vi "BuildExperiment.vi"(0 "object in":refnum<class "Application.lvclass">, 2 "Experiment Settings":T1={"Frequencies (MHz)"=[], "Camera Settings"={"Minimum Time between\n frames(s)"=10.0, "Number of Frames"=0}, "Flowrates (ul/min)"=[], "Voltages"=[]} {"Camera Settings"."Minimum Time between\n frames(s)" min=0.005}, 5 "error in (no error)":errorcluster) -> (14 "object out":refnum<class "Application.lvclass">, 19 "error out":errorcluster)   [LabVIEW 2023, in "Application.lvclass"]
uses:
  Application.lvclass
  Application.lvclass/Application.ctl
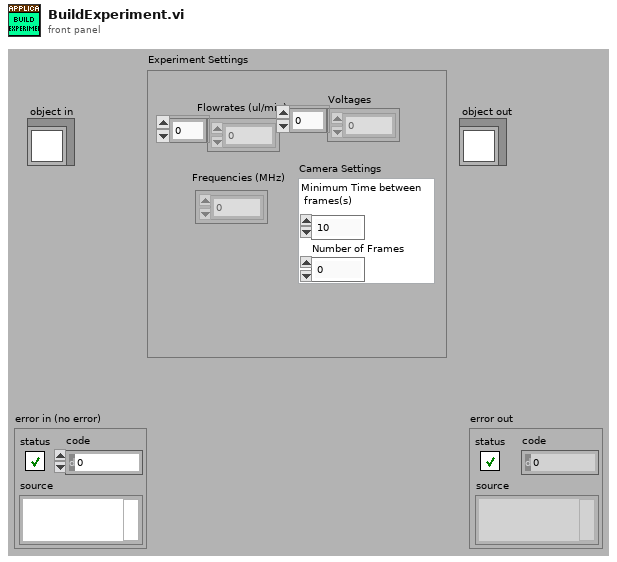
[diagram p1: front panel]
types:
  T1 = cluster{"Frequencies (MHz)":dbl[], "Camera Settings":cluster{"Minimum Time between\n frames(s)":dbl, "Number of Frames":i32}, "Flowrates (ul/min)":dbl[], "Voltages":dbl[]}
  T2 = cluster{"Minimum Time between\n frames(s)":dbl, "Number of Frames":i32}
  T3 = cluster{"Flowrates (ul/min)":dbl, "Voltages":dbl, "Numeric":dbl}
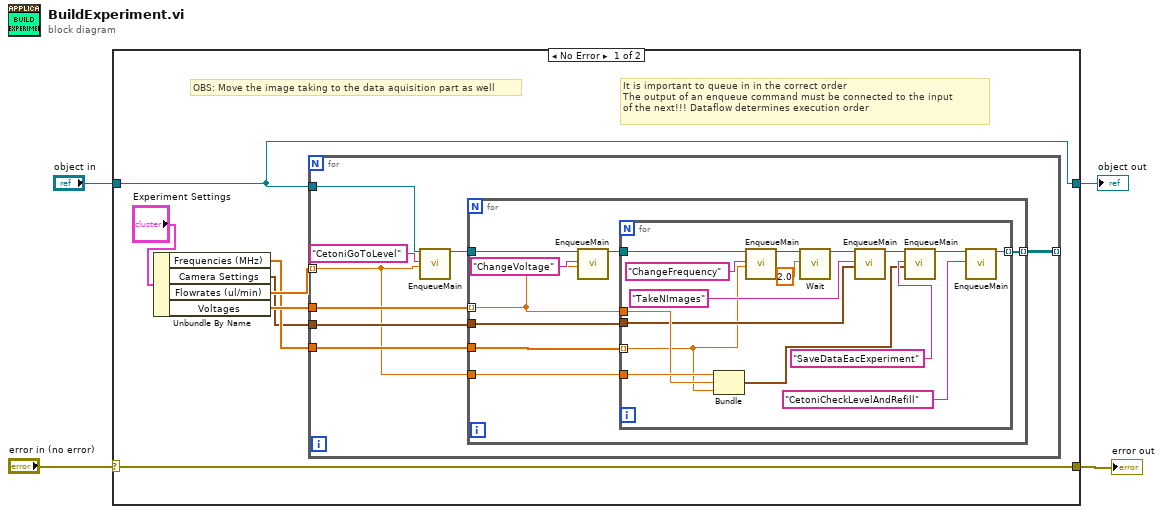
[diagram p0: block diagram]
diagram:
  n1 = case shown="No Error" "error in (no error)" {
    selector: "error in (no error)" -> [w11 w45]
    tunnel: [w11 w45] -> w3
    tunnel: [w10 w44] -> w1
    tunnel: "object in" -> [w10 w44]
    frame No Error {
      # "OBS: Move the image taking to the data aquisition part as well"
      # "It is important to queue in in the correct order\nThe output of an enqueue command must be connected to the input\nof the next!!! Dataflow determines execution order"
      n2 = Unbundle By Name("Experiment Settings") -> ("Frequencies (MHz)"=w6:dbl[], "Camera Settings"=w5:T2, "Flowrates (ul/min)"=w8:dbl[], "Voltages"=w7:dbl[])
      n3 = for {
        tunnel: w10 -> [w19]
        tunnel: [w16] -> _ mode=indexing
        tunnel: w8 -> [w12] mode=indexing
        tunnel: w7 -> [w15]
        tunnel: w6 -> [w14]
        tunnel: w5 -> [w13]
        n4 = call-dynamic "EnqueueMain.vi"("object in"=w19, "Message"="CetoniGoToLevel", "Message Data"=w12) -> ("object out"=w17:refnum<class "Application.lvclass">)  [unwired: 15 in, 1 out]
        n5 = for {
          tunnel: w17 -> [w25]
          tunnel: [w24] -> w16 mode=indexing
          tunnel: w15 -> [w20] mode=indexing
          tunnel: w14 -> [w23]
          tunnel: w13 -> [w22]
          tunnel: w12 -> [w21]
          n6 = call-dynamic "EnqueueMain.vi"("object in"=w25, "Message"="ChangeVoltage", "Message Data"=w20) -> ("object out"=w26:refnum<class "Application.lvclass">)  [unwired: 15 in, 1 out]
          n7 = for {
            tunnel: w26 -> [w40]
            tunnel: [w32] -> w24 mode=indexing
            tunnel: w23 -> [w35] mode=indexing
            tunnel: w22 -> [w36]
            tunnel: w21 -> [w38]
            tunnel: w20 -> [w37]
            n8 = Bundle("Flowrates (ul/min)"=w38, "Voltages"=w37, "Numeric"=w35) -> (w34:T3)  [unwired: 1 in]
            n9 = call-dynamic "EnqueueMain.vi"("object in"=w40, "Message"="ChangeFrequency", "Message Data"=w35) -> ("object out"=w30:refnum<class "Application.lvclass">)  [unwired: 15 in, 1 out]
            n10 = call-dynamic "Wait.vi"("object in"=w30, "Time to wait"=2.0) -> ("object out"=w29:refnum<class "Application.lvclass">)  [unwired: 15 in, 2 out]
            n11 = call-dynamic "EnqueueMain.vi"("object in"=w29, "Message"="TakeNImages", "Message Data"=w36) -> ("object out"=w39:refnum<class "Application.lvclass">)  [unwired: 15 in, 1 out]
            n12 = call-dynamic "EnqueueMain.vi"("object in"=w39, "Message"="SaveDataEacExperiment", "Message Data"=w34) -> ("object out"=w33:refnum<class "Application.lvclass">)  [unwired: 15 in, 1 out]
            n13 = call-dynamic "EnqueueMain.vi"("object in"=w33, "Message"="CetoniCheckLevelAndRefill") -> ("object out"=w32:refnum<class "Application.lvclass">)  [unwired: 16 in, 1 out]
          }
        }
      }
    }
    frame Error {
    }
  }
  "error out" <- w3
  "object out" <- w1
